vi "Running State Logic.vi"(8 "error in (no error)":errorcluster, 11 "CIFCorePlugin in":refnum<class "CIFCorePlugin.lvclass">) -> (0 "error out":errorcluster, 2 "Running State Logic":T1, 3 "CIFCorePlugin out":refnum<class "CIFCorePlugin.lvclass">)   [LabVIEW 2021, in "CIFCorePlugin.lvclass"]
uses:
  CIFCorePlugin.lvclass
  Typedef/Running State Logic.ctl
  CIFCorePlugin.lvclass/CIFCorePlugin.ctl
  CIFCoreCommon/Typedef/Plugin State.ctl
  CIFCoreCommon/CIFCoreCommon.lvlib
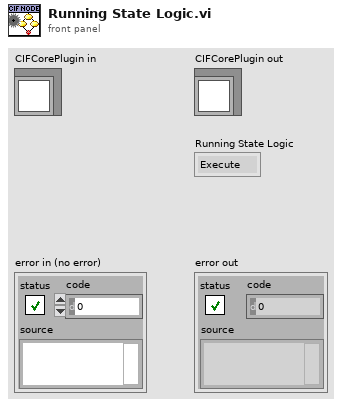
[diagram p1: front panel]
types:
  T1 = typedef "CIFCorePlugin.lvclass/Running State Logic.ctl" = enum16{"Execute", "Housekeep", "Cleanup", "Error", "Destroy"}
  T2 = typedef "CIFCorePlugin.lvclass/Energized States.ctl" = enum16{"Listen", "Prepare", "Execute", "Housekeep", "Cleanup", "Destroy"}
  T3 = typedef "CIFCoreCommon.lvlib/Plugin State.ctl" = enum32{"Null", "Creating", "Listening", "Running", "CleaningUp", "Destroying"}
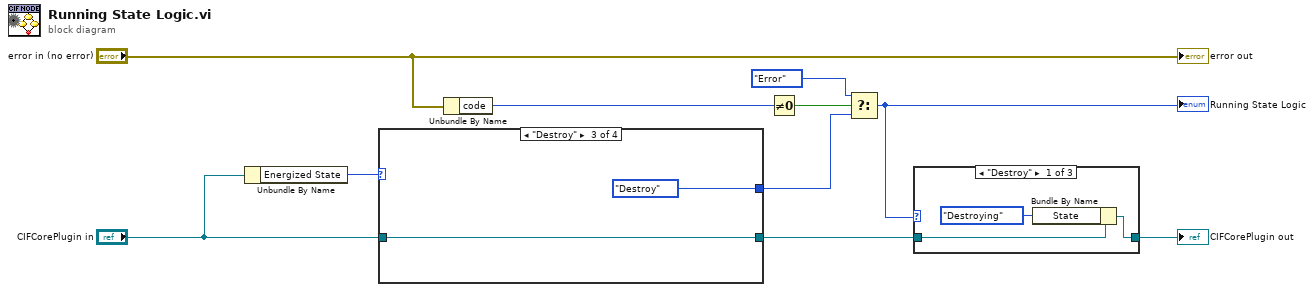
[diagram p0: block diagram]
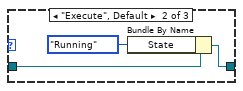
[diagram p2: hidden frame]
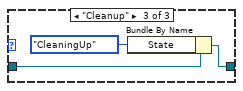
[diagram p3: hidden frame]
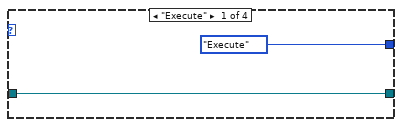
[diagram p4: hidden frame]
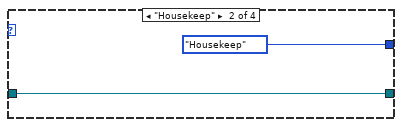
[diagram p5: hidden frame]
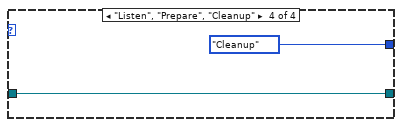
[diagram p6: hidden frame]
diagram:
  n1 = Unbundle By Name("CIFCorePlugin in") -> ("Energized State"=w7:T2)
  n2 = case shown="\"Destroy\"" w7 {
    tunnel: [Running_State_Logic."Execute" ("Execute State Logic") Running_State_Logic."Housekeep" ("Execute State Logic") Running_State_Logic."Destroy" ("Execute State Logic") Running_State_Logic."Cleanup" ("Execute State Logic")] -> w6
    tunnel: "CIFCorePlugin in" -> [w12 w14 w16 w18]
    tunnel: [w12 w14 w16 w18] -> w3
    frame "Execute" {
    }
    frame "Housekeep" {
    }
    frame "Destroy" {
    }
    frame "Listen", "Prepare", "Cleanup" {
    }
  }
  n3 = Unbundle By Name("error in (no error)") -> ("code"=w9:i32)
  n4 = Not Equal To 0?(x=w9) -> (x != 0?=w8:bool)
  n5 = Select(t=Running_State_Logic."Error" ("Execute State Logic"), s=w8, f=w6) -> (s? t:f=w1:T1)
  "Running State Logic" <- w1
  n6 = case shown="\"Destroy\"" w1 {
    tunnel: w3 -> [w20 w23 w26]
    tunnel: [w19 w22 w25] -> w2
    frame "Destroy" {
      n7 = Bundle By Name(cluster=w20, "State"=Plugin_State."Destroying" ("Status.State")) -> (w19:refnum<class "CIFCorePlugin.lvclass">)
    }
    frame "Execute", Default {
      n8 = Bundle By Name(cluster=w23, "State"=Plugin_State."Running" ("Status.State")) -> (w22:refnum<class "CIFCorePlugin.lvclass">)
    }
    frame "Cleanup" {
      n9 = Bundle By Name(cluster=w26, "State"=Plugin_State."CleaningUp" ("Status.State")) -> (w25:refnum<class "CIFCorePlugin.lvclass">)
    }
  }
  "CIFCorePlugin out" <- w2
  "error out" <- "error in (no error)"
